vi "Create Polar Plot.vi"() -> (0 "Polar Plot":picture)   [LabVIEW 2012]
doc: "Uses the Polar Graph VI to draw a polar plot in a picture indicator.\n\nNote: You must have the LabVIEW Full or Professional Development Systems to run this example."
panel:
  in  "Points":cluster{dbl, "start":dbl}[](array[cluster])=[{1.948739289613716, "start"=0.0}, {1.95208936739026, "start"=1.0}, {1.4279484317206041, "start"=2.0}, {1.7516994274248912, "start"=3.0}, {1.0500048691873245, "start"=4.0}, {1.3518656158711042, "start"=5.0}, {1.185027644133083, "start"=6.0}, {1.9097573856639853, "start"=7.0}, {1.8645203591510633, "start"=8.0}, {1.3833302078052867, "start"=9.0}, {1.51206650708947, "start"=10.0}, {1.5741987232711199, "start"=11.0}, {1.4380448815410523, "start"=12.0}, {1.8747290754422257, "start"=13.0}, {1.1472216873597243, "start"=14.0}, {1.4702701955405082, "start"=15.0}, {1.034125888391993, "start"=16.0}, {1.7901536559794615, "start"=17.0}, {1.5461543571110092, "start"=18.0}, {1.1251708677223853, "start"=19.0}, {1.3461841958807756, "start"=20.0}, {1.9853634738711334, "start"=21.0}, {1.8668776774460112, "start"=22.0}, {1.4803653198217546, "start"=23.0}, {1.9676827715154352, "start"=24.0}, {1.8770135366854634, "start"=25.0}, {1.6535830083623095, "start"=26.0}, {1.471506204376092, "start"=27.0}, {1.0379920716541609, "start"=28.0}, {1.2078043602209556, "start"=29.0}, {1.745255781445866, "start"=30.0}, {1.180082249644947, "start"=31.0}, {1.1678132590085208, "start"=32.0}, {1.630559105515402, "start"=33.0}, {1.0136291048861992, "start"=34.0}, {1.0934497484348427, "start"=35.0}, {1.1173233504672542, "start"=36.0}, {1.6576417802787793, "start"=37.0}, {1.0114477447507728, "start"=38.0}, {1.6657137312040453, "start"=39.0}, {1.4991441876857303, "start"=40.0}, {1.5027032553594801, "start"=41.0}, {1.2449073064535578, "start"=42.0}, {1.4066777241201436, "start"=43.0}, {1.2518633693399135, "start"=44.0}, {1.951153251175075, "start"=45.0}, {1.8708422987407662, "start"=46.0}, {1.5978340147134416, "start"=47.0}, {1.9627248327317708, "start"=48.0}, {1.0097962796681987, "start"=49.0}, {1.8646423694779626, "start"=50.0}, {1.884942650906524, "start"=51.0}, {1.6078367491264045, "start"=52.0}, {1.3141140710299062, "start"=53.0}, {1.1374502273860778, "start"=54.0}, {1.8565297511169936, "start"=55.0}, {1.9106279334432779, "start"=56.0}, {1.2842418555795307, "start"=57.0}, {1.7292694128726156, "start"=58.0}, {1.9434873825366616, "start"=59.0}, {1.6851631065444894, "start"=60.0}, {1.1236423693472868, "start"=61.0}, {1.2026817886394894, "start"=62.0}, {1.7590803974124227, "start"=63.0}, {1.5488120466948738, "start"=64.0}, {1.5404271337927624, "start"=65.0}, {1.6990374780748434, "start"=66.0}, {1.4431519201088934, "start"=67.0}, {1.6573324974228723, "start"=68.0}, {1.3907087252181414, "start"=69.0}, {1.2388583788006131, "start"=70.0}, {1.5639689962293617, "start"=71.0}, {1.4358296333418077, "start"=72.0}, {1.540652889660316, "start"=73.0}, {1.0477430439129067, "start"=74.0}, {1.9392891167422992, "start"=75.0}, {1.814435926416783, "start"=76.0}, {1.6150176737355086, "start"=77.0}, {1.711005658786246, "start"=78.0}, {1.3750485027144843, "start"=79.0}, {1.5308663380214675, "start"=80.0}, {1.0638338666262825, "start"=81.0}, {1.6053821906292494, "start"=82.0}, {1.8513764601993892, "start"=83.0}, {1.3060837797048057, "start"=84.0}, {1.743571249350328, "start"=85.0}, {1.526783005116488, "start"=86.0}, {1.8244213304782195, "start"=87.0}, {1.4589693204495249, "start"=88.0}, {1.6602118241247292, "start"=89.0}, {1.6111816193996067, "start"=90.0}, {1.3955553234863398, "start"=91.0}, {1.3749605867465005, "start"=92.0}, {1.9949569414300392, "start"=93.0}, {1.5599650153671951, "start"=94.0}, {1.581392728081621, "start"=95.0}, {1.5088193181335534, "start"=96.0}, {1.5668540154097195, "start"=97.0}, {1.0440018210672397, "start"=98.0}, {1.9484349278947612, "start"=99.0}, {1.3705795632638038, "start"=100.0}, {1.3639802111464006, "start"=101.0}, {1.3182706132729176, "start"=102.0}, {1.8402439741281875, "start"=103.0}, {1.3253616488424702, "start"=104.0}, {1.825816502170822, "start"=105.0}, {1.7497057568856111, "start"=106.0}, {1.5825281578049681, "start"=107.0}, {1.6920536308962522, "start"=108.0}, {1.2611120125633728, "start"=109.0}, {1.7120041166632967, "start"=110.0}, {1.8267722607874983, "start"=111.0}, {1.2163452119898777, "start"=112.0}, {1.9323140994315278, "start"=113.0}, {1.4172747546105802, "start"=114.0}, {1.3182766499895497, "start"=115.0}, {1.8896191107350426, "start"=116.0}, {1.9743565088379933, "start"=117.0}, {1.658270883261264, "start"=118.0}, {1.3297344687771784, "start"=119.0}, {1.833811357734519, "start"=120.0}, {1.5252980960449676, "start"=121.0}, {1.4112647262559108, "start"=122.0}, {1.920350216349213, "start"=123.0}, {1.667493046097869, "start"=124.0}, {1.5441226661513296, "start"=125.0}, {1.2056926570801494, "start"=126.0}, {1.9220241431412817, "start"=127.0}, {1.322784341070224, "start"=128.0}, {1.2995893597970267, "start"=129.0}, {1.998046347462427, "start"=130.0}, {1.0366808960138996, "start"=131.0}, {1.9781670813917307, "start"=132.0}, {1.7373186556979687, "start"=133.0}, {1.4190618656178238, "start"=134.0}, {1.4452638336941737, "start"=135.0}, {1.2466070299804297, "start"=136.0}, {1.1659508032244255, "start"=137.0}, {1.2499023262105342, "start"=138.0}, {1.6777162394192648, "start"=139.0}, {1.3907252372636996, "start"=140.0}, {1.4452380983120905, "start"=141.0}, {1.5136270878292872, "start"=142.0}, {1.1295639112340579, "start"=143.0}, {1.3719722874873859, "start"=144.0}, {1.2005921557779249, "start"=145.0}, {1.489499683655443, "start"=146.0}, {1.0845769931438556, "start"=147.0}, {1.2993237154730424, "start"=148.0}, {1.2883380338570467, "start"=149.0}, {1.9912416460102182, "start"=150.0}, {1.468272226651219, "start"=151.0}, {1.2267875514026398, "start"=152.0}, {1.4454645028671949, "start"=153.0}, {1.1298509876768579, "start"=154.0}, {1.4049514174030988, "start"=155.0}, {1.284652227777868, "start"=156.0}, {1.0107792125543984, "start"=157.0}, {1.5520830994842654, "start"=158.0}, {1.1695247902871784, "start"=159.0}, {1.6265049531287374, "start"=160.0}, {1.9241326893755892, "start"=161.0}, {1.5449987938472685, "start"=162.0}, {1.6424456505814053, "start"=163.0}, {1.6026103990994098, "start"=164.0}, {1.2909625313159374, "start"=165.0}, {1.0250818168753897, "start"=166.0}, {1.1517129727688653, "start"=167.0}, {1.896696027066237, "start"=168.0}, {1.5273142772213737, "start"=169.0}, {1.4757011468148742, "start"=170.0}, {1.974834170107397, "start"=171.0}, {1.1126063277481162, "start"=172.0}, {1.1260962171558309, "start"=173.0}, {1.4789804709337337, "start"=174.0}, {1.447613936304909, "start"=175.0}, {1.6307059160158637, "start"=176.0}, {1.476301882314637, "start"=177.0}, {1.1445828809718979, "start"=178.0}, {1.8256134922537035, "start"=179.0}] {"start" format="%0.2f"; "?" format="%0.2f"}
  in  "polar attributes":T1={"maximum"=2.0, "minimum"=0.0, "clip to min"=FALSE, "log"=FALSE, "grid color"=3381657, "plot color"=16711680, "fmt and prec"={"format"=enum."Decimal", "precision"=2}, "visible section"=4} {"minimum" format="%0.2f"; "maximum" format="%0.2f"}
  in  "desired font":T2(ring)=enum."Application Font"
  in  "user-specified font":T3={"Font Name:"="monaco", "Size"=9, "Strikeout?"=FALSE, "Italic?"=FALSE, "Underline?"=FALSE, "Outline?"=FALSE, "Shadow?"=FALSE, "Bold?"=FALSE}
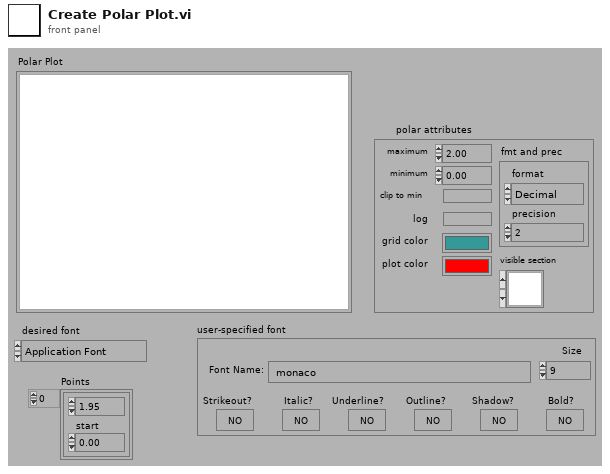
[diagram p1: front panel]
types:
  T1 = cluster{"maximum":dbl, "minimum":dbl, "clip to min":bool, "log":bool, "grid color":u32, "plot color":u32, "fmt and prec":cluster{"format":enum8{"Decimal", "Scientific", "Engineering", "Binary", "Octal", "Hex"}, "precision":u8}, "visible section":u16}
  T2 = enum16{"User-specified Font", "Application Font", "System Font", "Dialog Font"}
  T3 = cluster{"Font Name:":string, "Size":i16, "Strikeout?":bool, "Italic?":bool, "Underline?":bool, "Outline?":bool, "Shadow?":bool, "Bold?":bool}
  T4 = typedef "LVBoundsTypeDef.ctl" = cluster{"Width":u32, "Height":u32}
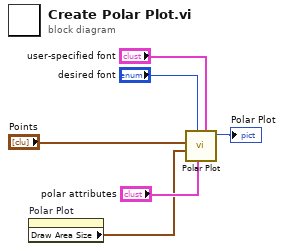
[diagram p0: block diagram]
diagram:
  n1 = property on="Polar Plot" class="Pict"() -> ("Draw Area Size"=w2:T4)  [unwired: 2 in, 2 out]
  n2 = call <vilib>:"Polar Plot.vi"("[user-specified font]"="user-specified font", "polar attributes"="polar attributes", "desired font(Application)"="desired font", "dimensions (w,h)"=w2, "data array [mag, phase (deg)]"="Points") -> ("new picture"=→"Polar Plot":picture)  [unwired: 1 in, 5 out]
